vi "Camera_Config_Specific_Attributes.vi"(4 "Crop?":bool, 5 "Camera":T1, 6 "Detect Movement":bool, 8 "error in (no error)":errorcluster, 10 "Refnum in":T2, 11 "input cluster":T3={"Pinch-valve"="", "XLP 6000 Pump"="", "Camera1"="", "Camera2"="", "Img_Capt"=FALSE, "Actuator"=FALSE, "Pump"=FALSE, "Cam 1"=FALSE, "Cam 2"=FALSE, "Empty_Refill"=FALSE, "Crop"=FALSE, "Light intensity"=0, "Exposure Time"=0.0, "Sample Name"="", "Operator"="", "Calibration 1"=path "", "Calibration 2"=path "", "Framerate"=0, "Timeout Sample"=0, "Collection date"="", "Sample size threshold"=0, "Empty start"=0, "Command"="", "Station"="", "Species Name"="", "Other Notes"="", "Aperture"=enum."Item 0", "Image Process Queue Size"=0, "Image Save Queue Size"=0, "Overload threshold"=0, "Max Framerate"=0, "Rectangle 1"={"Left"=0, "Top"=0, "Right"=0, "Bottom"=0, "Rotation"=0.0}, "Rectangle 2"={"Left"=0, "Top"=0, "Right"=0, "Bottom"=0, "Rotation"=0.0}, "Detection Region %"=200.0, "Detect 1"=path "", "Detect 2"=path "", "Max large object threshold"=500, "Open(T)/Close(F)"=FALSE, "Img_Capt Begin"=FALSE, "Dispense Speed"=0, "Flush Size"=0, "Location"="", "Latitude"="", "Longitude"="", "Determiner"="", "Sex"="", "Camera1_Img"=refnum, "Camera2_Img"=refnum, "Img1_Orig_Disp"=refnum, "Img2_Orig_Disp"=refnum, "Img1_Orig_RGB"=refnum, "Img2_Orig_RGB"=refnum, "Blue_Plane_Extract"=refnum, "Subtracted_Plane"=refnum, "Img1_Binary"=refnum, "Img2_Binary"=refnum, "Crop_Mask"=refnum, "Img1_Save"=refnum, "Img2_Save"=refnum, "Img1_Cali_Full"=refnum, "Img2_Cali_Full"=refnum, "Img1_Cali_Detect"=refnum, "Img2_Cali_Detect"=refnum, "Cam 1 queue"=refnum, "Cam 2 queue"=refnum, "Cam 1 - save queue"=refnum, "Cam 2 - save queue"=refnum, "Overlay_Ring"=0, "SystemVersion"=0, "System Serial"="", "Legacy Cam Attributes"=FALSE, "Camera Orientation 1"="", "Camera Orientation 2"="", "Pixel to mm 1"=0.0, "Pixel to mm 2"=0.0, "CAM1 Model"=enum."a2A5328-15ucBAS", "CAM2 Model"=enum."a2A5328-15ucBAS"} {"SystemVersion" items=["Standard", "XL"]; "Overlay_Ring" items=["Session Data", "Extended Setup", "Buffer", "Camera", "Dispenser", "Stats", "Connections"]; "Flush Size" min=1; "Dispense Speed" min=1; "Rectangle 2"."Rotation" format="%.2f"; "Rectangle 2"."Left" scale=0.0..1024.0; "Rectangle 2"."Right" scale=0.0..1024.0; "Rectangle 1"."Rotation" format="%.2f"; "Rectangle 1"."Left" scale=0.0..1024.0; "Rectangle 1"."Right" scale=0.0..1024.0; "Max Framerate" min=1; "Overload threshold" min=1; "Image Save Queue Size" min=1; "Image Process Queue Size" min=1; "Empty start" min=1; "Sample size threshold" min=1; "Framerate" min=1; "Light intensity" scale=0.0..100.0}) -> (0 "error out":errorcluster, 3 "Refnum out":T2)   [LabVIEW 2022 SP3]
uses:
  <vilib>/userdefined/High Color/IMAQdx.ctl
  controls/Data.ctl
  <vilib>/vision/Image Controls.llb/IMAQ Image.ctl
  Camera_ID.ctl
  <resource>/objmgr/imaqdx.rc
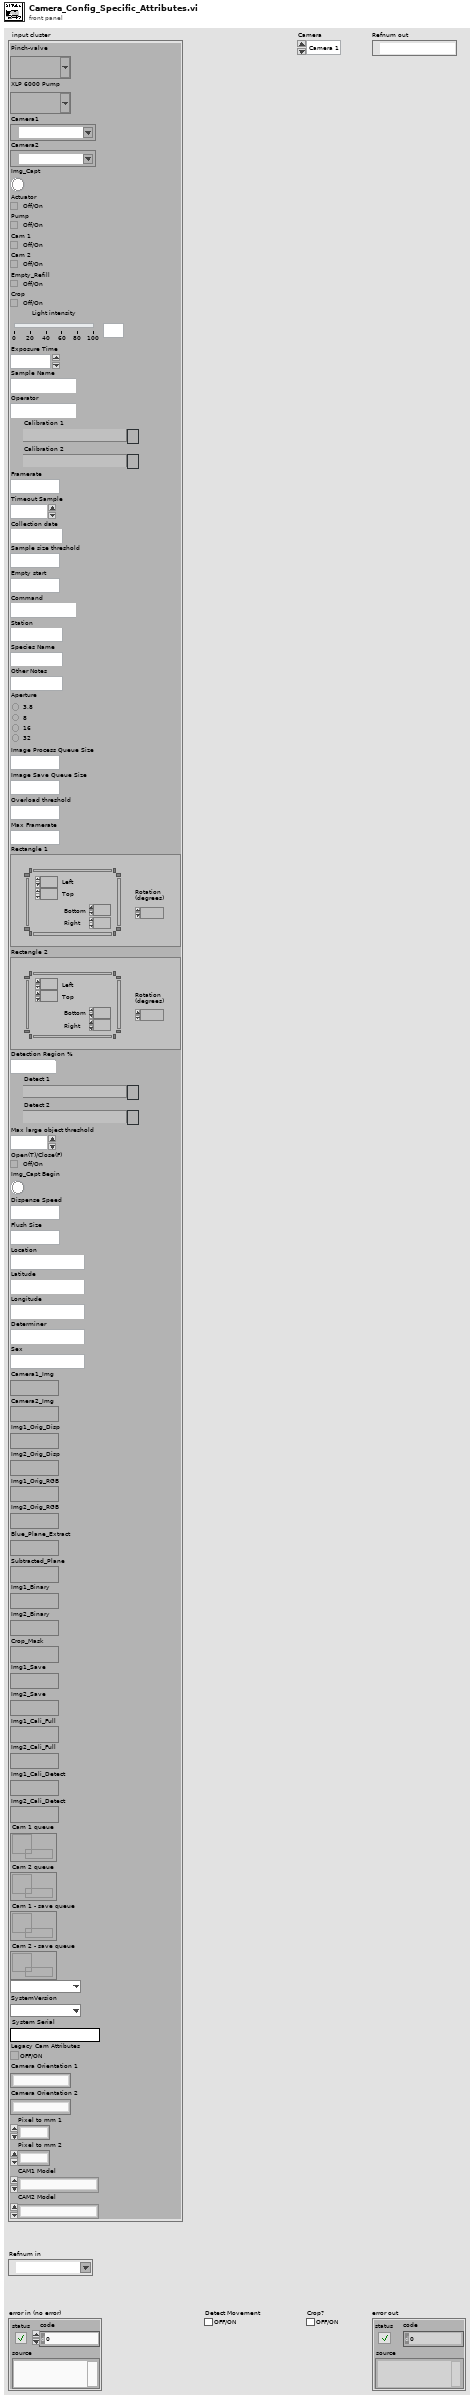
[diagram p1: front panel]
types:
  T1 = typedef "Camera_ID.ctl" = enum16{"Camera 1", "Camera 2"}
  T2 = typedef "IMAQdx.ctl" = refnum<k21>
  T3 = typedef "Data.ctl" = cluster{"Pinch-valve":refnum<visa-resource-name>, "XLP 6000 Pump":refnum<visa-resource-name>, "Camera1":T2, "Camera2":T2, "Img_Capt":bool, "Actuator":bool, "Pump":bool, "Cam 1":bool, "Cam 2":bool, "Empty_Refill":bool, "Crop":bool, "Light intensity":i32, "Exposure Time":dbl, "Sample Name":string, "Operator":string, "Calibration 1":path, "Calibration 2":path, "Framerate":i32, "Timeout Sample":i32, "Collection date":string, "Sample size threshold":i32, "Empty start":u32, "Command":string, "Station":string, "Species Name":string, "Other Notes":string, "Aperture":enum32{"Item 0", "Item 1", "Item 2", "Item 3"}, "Image Process Queue Size":i32, "Image Save Queue Size":i32, "Overload threshold":i32, "Max Framerate":i32, "Rectangle 1":T4, "Rectangle 2":T4, "Detection Region %":dbl, "Detect 1":path, "Detect 2":path, "Max large object threshold":i32, "Open(T)/Close(F)":bool, "Img_Capt Begin":bool, "Dispense Speed":i32, "Flush Size":i32, "Location":string, "Latitude":string, "Longitude":string, "Determiner":string, "Sex":string, "Camera1_Img":T5, "Camera2_Img":T5, "Img1_Orig_Disp":T5, "Img2_Orig_Disp":T5, "Img1_Orig_RGB":T5, "Img2_Orig_RGB":T5, "Blue_Plane_Extract":T5, "Subtracted_Plane":T5, "Img1_Binary":T5, "Img2_Binary":T5, "Crop_Mask":T5, "Img1_Save":T5, "Img2_Save":T5, "Img1_Cali_Full":T5, "Img2_Cali_Full":T5, "Img1_Cali_Detect":T5, "Img2_Cali_Detect":T5, "Cam 1 queue":refnum<queue>, "Cam 2 queue":refnum<queue>, "Cam 1 - save queue":refnum<queue>, "Cam 2 - save queue":refnum<queue>, "Overlay_Ring":u16, "SystemVersion":u16, "System Serial":string, "Legacy Cam Attributes":bool, "Camera Orientation 1":string, "Camera Orientation 2":string, "Pixel to mm 1":dbl, "Pixel to mm 2":dbl, "CAM1 Model":enum16{"a2A5328-15ucBAS", "acA1920-155uc"}, "CAM2 Model":enum16{"a2A5328-15ucBAS", "acA1920-155uc"}}
  T4 = typedef "IMAQ Rectangle" = cluster{"Left":i32, "Top":i32, "Right":i32, "Bottom":i32, "Rotation":dbl}
  T5 = typedef "IMAQ Image.ctl" = refnum<image>
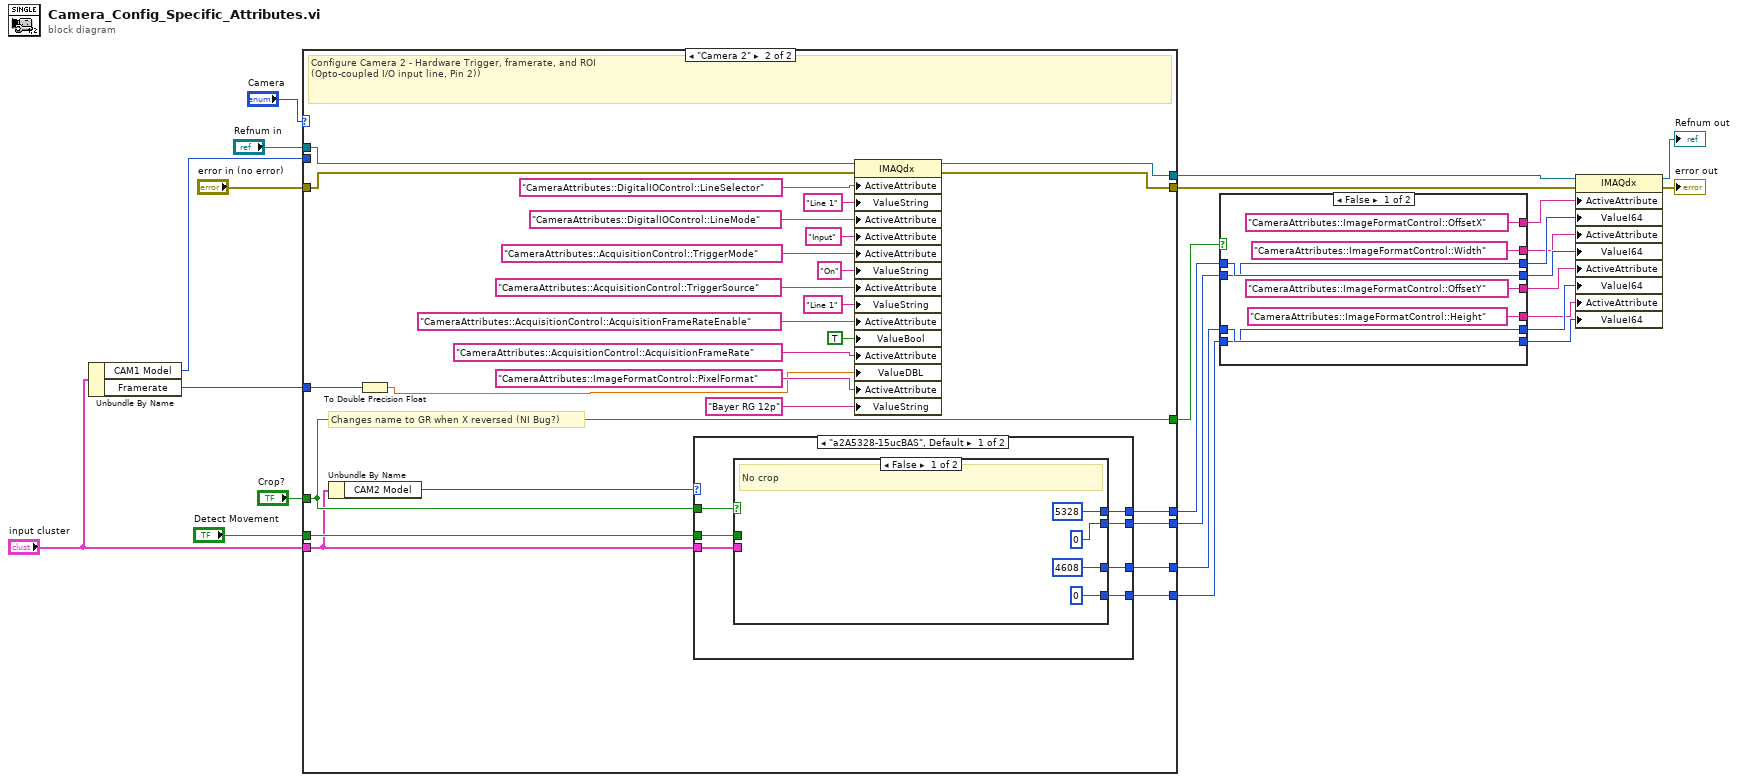
[diagram p0: block diagram]
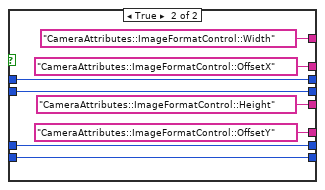
[diagram p2: hidden frame]
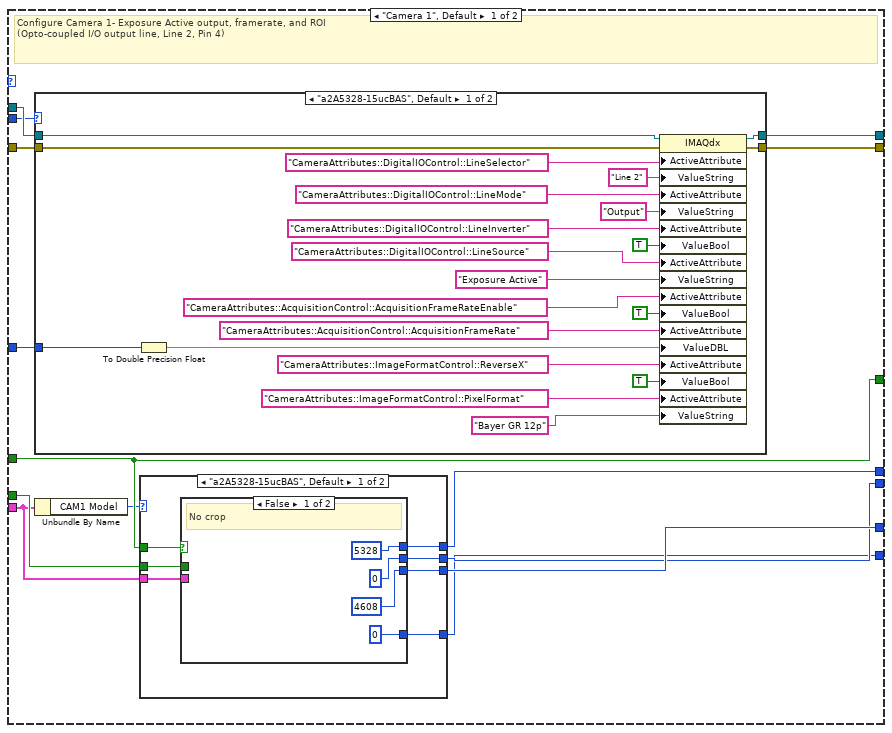
[diagram p3: hidden frame]
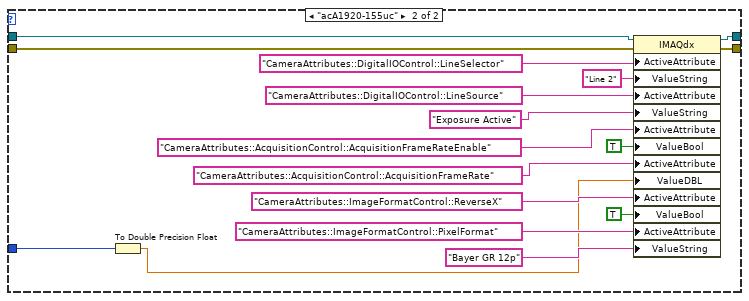
[diagram p4: hidden frame]
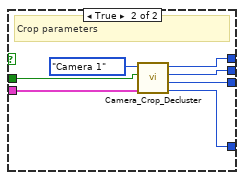
[diagram p5: hidden frame]
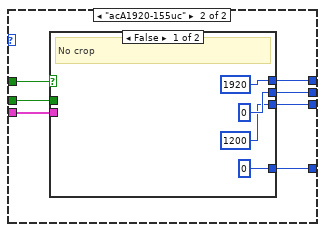
[diagram p6: hidden frame]
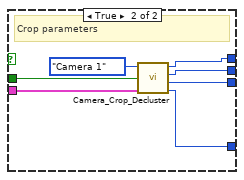
[diagram p7: hidden frame]
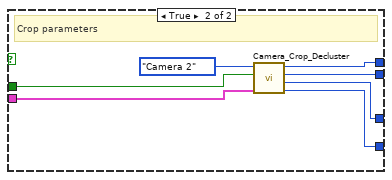
[diagram p8: hidden frame]
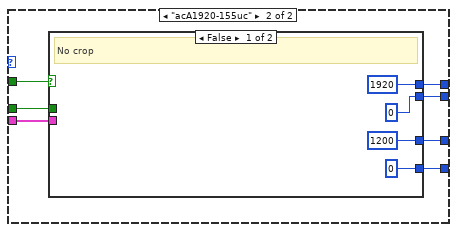
[diagram p9: hidden frame]
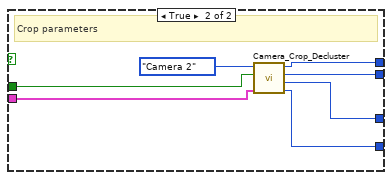
[diagram p10: hidden frame]
diagram:
  n1 = Unbundle By Name("input cluster") -> ("CAM1 Model"=w1:enum16{"a2A5328-15ucBAS", "acA1920-155uc"}, "Framerate"=w2:i32)
  n2 = case shown="\"Camera 2\"" "Camera" {
    tunnel: "Refnum in" -> [w39 w133]
    tunnel: [w38 w132] -> w12
    tunnel: [w37 w131] -> w5
    tunnel: w2 -> [w29 w120]
    tunnel: [w35 w140] -> w18
    tunnel: [w36 w139] -> w15
    tunnel: [w33 w137] -> w20
    tunnel: [w34 w138] -> w16
    tunnel: "Crop?" -> [w32 w136]
    tunnel: [w32 w136] -> w13
    tunnel: "input cluster" -> [w28 w122]
    tunnel: "Detect Movement" -> [w31 w135]
    tunnel: "error in (no error)" -> [w30 w130]
    tunnel: w1 -> [w26 _]
    frame "Camera 1", Default {
      # "Configure Camera 1- Exposure Active output, framerate, and ROI\n(Opto-coupled I/O output line, Line 2, Pin 4)"
      n3 = case shown="\"a2A5328-15ucBAS\", Default" w26 {
        tunnel: w39 -> [w60 w77]
        tunnel: [w58 w76] -> w38
        tunnel: [w57 w75] -> w37
        tunnel: w30 -> [w59 w73]
        tunnel: w29 -> [w46 w62]
        frame "a2A5328-15ucBAS", Default {
          n4 = To Double Precision Float(number=w46) -> (double precision float=w45:dbl)
          n5 = property class="IMAQdx"(reference=w60, error in=w59, "ActiveAttribute"="CameraAttributes::DigitalIOControl::LineSelector", "ValueString"="Line 2", "ActiveAttribute"="CameraAttributes::DigitalIOControl::LineMode", "ValueString"="Output", "ActiveAttribute"="CameraAttributes::DigitalIOControl::LineInverter", "ValueBool"=TRUE, "ActiveAttribute"="CameraAttributes::DigitalIOControl::LineSource", "ValueString"="Exposure Active", "ActiveAttribute"="CameraAttributes::AcquisitionControl::AcquisitionFrameRateEnable", "ValueBool"=TRUE, "ActiveAttribute"="CameraAttributes::AcquisitionControl::AcquisitionFrameRate", "ValueDBL"=w45, "ActiveAttribute"="CameraAttributes::ImageFormatControl::ReverseX", "ValueBool"=TRUE, "ActiveAttribute"="CameraAttributes::ImageFormatControl::PixelFormat", "ValueString"="Bayer GR 12p") -> (reference out=w58:T2, error out=w57:errorcluster)
        }
        frame "acA1920-155uc" {
          n6 = To Double Precision Float(number=w62) -> (double precision float=w61:dbl)
          n7 = property class="IMAQdx"(reference=w77, error in=w73, "ActiveAttribute"="CameraAttributes::DigitalIOControl::LineSelector", "ValueString"="Line 2", "ActiveAttribute"="CameraAttributes::DigitalIOControl::LineSource", "ValueString"="Exposure Active", "ActiveAttribute"="CameraAttributes::AcquisitionControl::AcquisitionFrameRateEnable", "ValueBool"=TRUE, "ActiveAttribute"="CameraAttributes::AcquisitionControl::AcquisitionFrameRate", "ValueDBL"=w61, "ActiveAttribute"="CameraAttributes::ImageFormatControl::ReverseX", "ValueBool"=TRUE, "ActiveAttribute"="CameraAttributes::ImageFormatControl::PixelFormat", "ValueString"="Bayer GR 12p") -> (reference out=w76:T2, error out=w75:errorcluster)
        }
      }
      n8 = Unbundle By Name(w28) -> ("CAM1 Model"=w27:enum16{"a2A5328-15ucBAS", "acA1920-155uc"})
      n9 = case shown="\"a2A5328-15ucBAS\", Default" w27 {
        tunnel: [w81 w102] -> w36
        tunnel: [w79 w101] -> w35
        tunnel: [w80 w100] -> w34
        tunnel: [w78 w99] -> w33
        tunnel: w32 -> [w84 w98]
        tunnel: w28 -> [w82 w97]
        tunnel: w31 -> [w83 w96]
        frame "a2A5328-15ucBAS", Default {
          n10 = case shown="False" w84 {
            tunnel: [5328 w94] -> w81
            tunnel: [4608 w92] -> w79
            tunnel: [i64 0 w93] -> w80
            tunnel: [0 w91] -> w78
            tunnel: w82 -> [_ w90]
            tunnel: w83 -> [_ w89]
            frame False {
              # "No crop"
            }
            frame True {
              # "Crop parameters"
              n11 = call "Camera_Crop_Decluster.vi"("input cluster"=w90, "Detect Movement"=w89, "Camera"=Camera_ID."Camera 1") -> ("OffsetY"=w91:i64, "Height"=w92:i64, "OffsetX"=w93:i64, "Width"=w94:i64)  [unwired: 5 in]
            }
          }
        }
        frame "acA1920-155uc" {
          n12 = case shown="False" w98 {
            tunnel: [i64 1920 w112] -> w102
            tunnel: [1200 w110] -> w101
            tunnel: [i64 0 w111] -> w100
            tunnel: [0 w109] -> w99
            tunnel: w97 -> [_ w108]
            tunnel: w96 -> [_ w107]
            frame False {
              # "No crop"
            }
            frame True {
              # "Crop parameters"
              n13 = call "Camera_Crop_Decluster.vi"("input cluster"=w108, "Detect Movement"=w107, "Camera"=Camera_ID."Camera 1") -> ("OffsetY"=w109:i64, "Height"=w110:i64, "OffsetX"=w111:i64, "Width"=w112:i64)  [unwired: 5 in]
            }
          }
        }
      }
    }
    frame "Camera 2" {
      # "Changes name to GR when X reversed (NI Bug?)"
      # "Configure Camera 2 - Hardware Trigger, framerate, and ROI \n(Opto-coupled I/O input line, Pin 2))"
      n14 = Unbundle By Name(w122) -> ("CAM2 Model"=w121:enum16{"a2A5328-15ucBAS", "acA1920-155uc"})
      n15 = To Double Precision Float(number=w120) -> (double precision float=w119:dbl)
      n16 = case shown="\"a2A5328-15ucBAS\", Default" w121 {
        tunnel: [w142 w165] -> w140
        tunnel: [w144 w164] -> w139
        tunnel: [w143 w163] -> w138
        tunnel: [w141 w162] -> w137
        tunnel: w136 -> [w147 w161]
        tunnel: w122 -> [w146 w160]
        tunnel: w135 -> [w145 w159]
        frame "a2A5328-15ucBAS", Default {
          n17 = case shown="False" w147 {
            tunnel: [i64 4608 w154] -> w142
            tunnel: [i64 5328 w156] -> w144
            tunnel: [i64 0 w155] -> w143
            tunnel: [i64 0 w153] -> w141
            tunnel: w146 -> [_ w158]
            tunnel: w145 -> [_ w152]
            frame False {
              # "No crop"
            }
            frame True {
              # "Crop parameters"
              n18 = call "Camera_Crop_Decluster.vi"("input cluster"=w158, "Detect Movement"=w152, "Camera"=Camera_ID."Camera 2") -> ("OffsetY"=w153:i64, "Height"=w154:i64, "OffsetX"=w155:i64, "Width"=w156:i64)  [unwired: 5 in]
            }
          }
        }
        frame "acA1920-155uc" {
          n19 = case shown="False" w161 {
            tunnel: [i64 1200 w172] -> w165
            tunnel: [i64 1920 w174] -> w164
            tunnel: [i64 0 w173] -> w163
            tunnel: [i64 0 w171] -> w162
            tunnel: w160 -> [_ w176]
            tunnel: w159 -> [_ w170]
            frame False {
              # "No crop"
            }
            frame True {
              # "Crop parameters"
              n20 = call "Camera_Crop_Decluster.vi"("input cluster"=w176, "Detect Movement"=w170, "Camera"=Camera_ID."Camera 2") -> ("OffsetY"=w171:i64, "Height"=w172:i64, "OffsetX"=w173:i64, "Width"=w174:i64)  [unwired: 5 in]
            }
          }
        }
      }
      n21 = property class="IMAQdx"(reference=w133, error in=w130, "ActiveAttribute"="CameraAttributes::DigitalIOControl::LineSelector", "ValueString"="Line 1", "ActiveAttribute"="CameraAttributes::DigitalIOControl::LineMode", "ActiveAttribute"="Input", "ActiveAttribute"="CameraAttributes::AcquisitionControl::TriggerMode", "ValueString"="On", "ActiveAttribute"="CameraAttributes::AcquisitionControl::TriggerSource", "ValueString"="Line 1", "ActiveAttribute"="CameraAttributes::AcquisitionControl::AcquisitionFrameRateEnable", "ValueBool"=TRUE, "ActiveAttribute"="CameraAttributes::AcquisitionControl::AcquisitionFrameRate", "ValueDBL"=w119, "ActiveAttribute"="CameraAttributes::ImageFormatControl::PixelFormat", "ValueString"="Bayer RG 12p") -> (reference out=w132:T2, error out=w131:errorcluster)
    }
  }
  n22 = case shown="False" w13 {
    tunnel: ["CameraAttributes::ImageFormatControl::Height" ("ActiveAttribute") "CameraAttributes::ImageFormatControl::OffsetY" ("ActiveAttribute")] -> w6
    tunnel: ["CameraAttributes::ImageFormatControl::OffsetY" ("ActiveAttribute") "CameraAttributes::ImageFormatControl::Height" ("ActiveAttribute")] -> w7
    tunnel: ["CameraAttributes::ImageFormatControl::Width" ("ActiveAttribute") "CameraAttributes::ImageFormatControl::OffsetX" ("ActiveAttribute")] -> w8
    tunnel: ["CameraAttributes::ImageFormatControl::OffsetX" ("ActiveAttribute") "CameraAttributes::ImageFormatControl::Width" ("ActiveAttribute")] -> w9
    tunnel: [w179 w188] -> w14
    tunnel: w15 -> [w180 w188]
    tunnel: w16 -> [w179 w187]
    tunnel: [w180 w187] -> w17
    tunnel: w18 -> [w178 w186]
    tunnel: [w177 w186] -> w19
    tunnel: w20 -> [w177 w185]
    tunnel: [w178 w185] -> w21
    frame False {
    }
    frame True {
    }
  }
  n23 = property class="IMAQdx"(reference=w12, error in=w5, "ActiveAttribute"=w9, "ValueI64"=w14, "ActiveAttribute"=w8, "ValueI64"=w17, "ActiveAttribute"=w7, "ValueI64"=w19, "ActiveAttribute"=w6, "ValueI64"=w21) -> (reference out=→"Refnum out":T2, error out=→"error out":errorcluster)
